vi "DAQ_DAQNodeConfigs.vi"(8 "error in":errorcluster, 10 "StreamCluster_TypeDef in":T1={"DAQ"={"ManagmentRate_Hz"=1000, "StreamRate_Hz"=10, "refDesArray"=[], "StreamRate_ms"=0, "ManagmentRate_ms"=1000}, "Modules"=[]}, 11 "DOM document in":refnum<k20>) -> (0 "error out":errorcluster={"status"=TRUE, "code"=-2633, "source"="Property Node (arg 1) in NI_XML.lvlib:Get Node Text Content.vi->CTR_ControlNodeConfigs.vi->CTR_ReadXML_Config.vi->CTRnode.vi"}, 2 "StreamCluster_TypeDef out":T1={"DAQ"={"ManagmentRate_Hz"=1000, "StreamRate_Hz"=10, "refDesArray"=[], "StreamRate_ms"=0, "ManagmentRate_ms"=1000}, "Modules"=[]}, 3 "DOM document out":refnum<k20>)   [LabVIEW 2024]
uses:
  Control/StreamCluster_TypeDef.ctl
  <vilib>/xml/Close Reference(Node).vi
  <vilib>/xml/NI_XML.lvlib
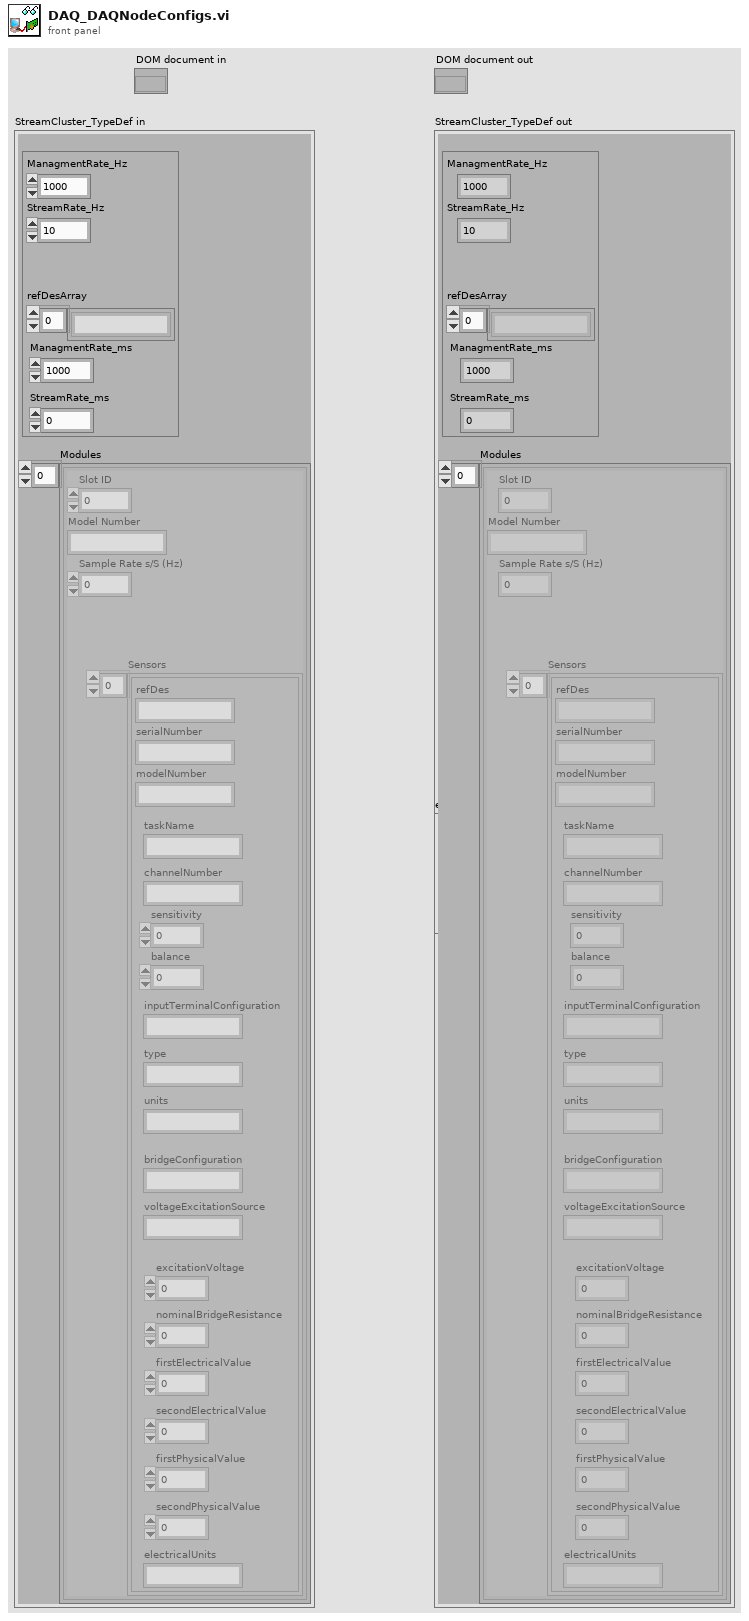
[diagram p1: front panel]
types:
  T1 = typedef "StreamCluster_TypeDef.ctl" = cluster{"DAQ":cluster{"ManagmentRate_Hz":i32, "StreamRate_Hz":i32, "refDesArray":string[], "StreamRate_ms":i32, "ManagmentRate_ms":i32}, "Modules":cluster{"Slot ID":i32, "Model Number":string, "Sample Rate s/S (Hz)":dbl, "Sensors":cluster{"refDes":string, "serialNumber":string, "modelNumber":string, "units":string, "balance":dbl, "sensitivity":dbl, "type":string, "inputTerminalConfiguration":string, "channelNumber":string, "taskName":string, "bridgeConfiguration":string, "excitationVoltage":dbl, "voltageExcitationSource":string, "nominalBridgeResistance":dbl, "firstElectricalValue":dbl, "secondElectricalValue":dbl, "firstPhysicalValue":dbl, "secondPhysicalValue":dbl, "electricalUnits":string}[]}[]}
  T2 = typedef "streamIO_states.ctl" = enum16{"Fault", "Initialize", "Stream", "Close"}
  T3 = cluster{"stream state":T2, "DAQ Node ID":i32, "Modules":cluster{"Slot ID":i32, "Model Number":string, "Sample Rate s/S (Hz)":dbl, "Sensors":cluster{"refDes":string, "serialNumber":string, "modelNumber":string, "units":string, "balance":dbl, "sensitivity":dbl, "type":string, "inputTerminalConfiguration":string, "channelNumber":string, "taskName":string, "bridgeConfiguration":string, "excitationVoltage":dbl, "voltageExcitationSource":string, "nominalBridgeResistance":dbl, "firstElectricalValue":dbl, "secondElectricalValue":dbl, "firstPhysicalValue":dbl, "secondPhysicalValue":dbl, "electricalUnits":string}[]}[], "DAQ IP Addr":string, "Restart":bool, "writer endpoint":refnum<k21>, "reader endpoint":refnum<k21>}[]
  T4 = cluster{"stream state":T2, "DAQ Node ID":i32, "Modules":cluster{"Slot ID":i32, "Model Number":string, "Sample Rate s/S (Hz)":dbl, "Sensors":cluster{"refDes":string, "serialNumber":string, "modelNumber":string, "units":string, "balance":dbl, "sensitivity":dbl, "type":string, "inputTerminalConfiguration":string, "channelNumber":string, "taskName":string, "bridgeConfiguration":string, "excitationVoltage":dbl, "voltageExcitationSource":string, "nominalBridgeResistance":dbl, "firstElectricalValue":dbl, "secondElectricalValue":dbl, "firstPhysicalValue":dbl, "secondPhysicalValue":dbl, "electricalUnits":string}[]}[], "DAQ IP Addr":string, "Restart":bool, "writer endpoint":refnum<k21>, "reader endpoint":refnum<k21>}
  T5 = cluster{"[0]":string, "[1]":string, "[2]":string, "[3]":string, "[4]":string, "[5]":string, "[6]":string, "[7]":string, "[8]":string}
  T6 = cluster{"Slot ID":i32, "Model Number":string, "Sample Rate s/S (Hz)":dbl, "Sensors":cluster{"refDes":string, "serialNumber":string, "modelNumber":string, "units":string, "balance":dbl, "sensitivity":dbl, "type":string, "inputTerminalConfiguration":string, "channelNumber":string, "taskName":string, "bridgeConfiguration":string, "excitationVoltage":dbl, "voltageExcitationSource":string, "nominalBridgeResistance":dbl, "firstElectricalValue":dbl, "secondElectricalValue":dbl, "firstPhysicalValue":dbl, "secondPhysicalValue":dbl, "electricalUnits":string}[]}[]
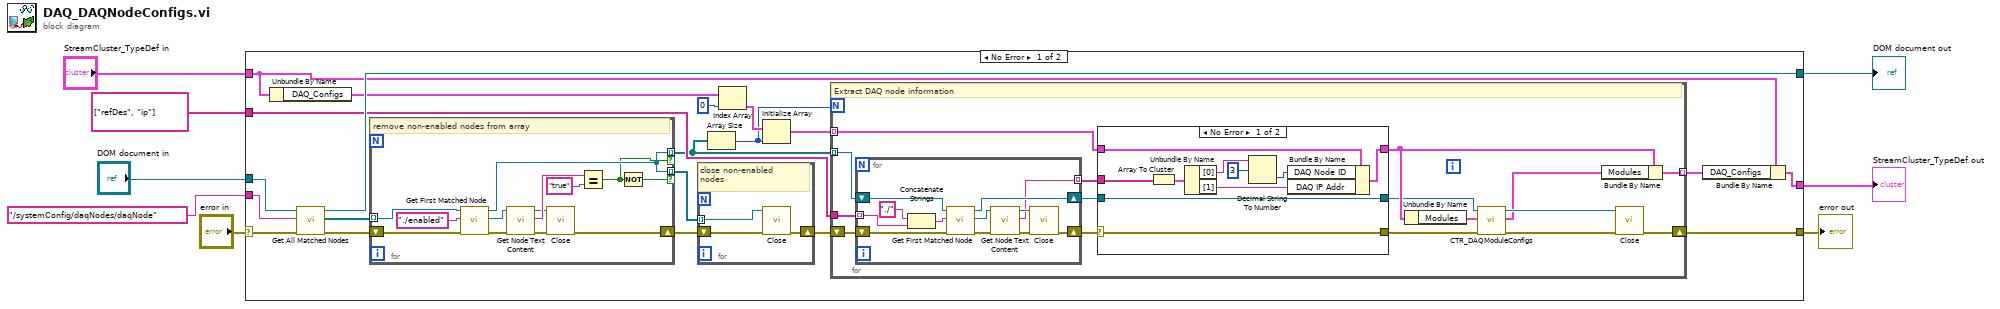
[diagram p0: block diagram]
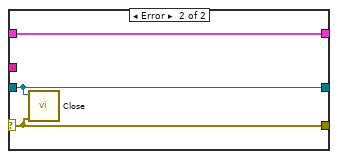
[diagram p2: hidden frame]
diagram:
  n1 = case shown="No Error" "error in" {
    selector: "error in" -> [w28 w88]
    tunnel: [w25 w88] -> w7
    tunnel: "StreamCluster_TypeDef in" -> [w24 w87]
    tunnel: [w23 w87] -> w5
    tunnel: "DOM document in" -> [w27 w86]
    tunnel: [w26 w86] -> w3
    tunnel: "/systemConfig/daqNodes/daqNode" ("XPath expression") -> [w14 _]
    tunnel: string[] ["refDes", "ip"] -> [w13 _]
    frame No Error {
      n2 = Unbundle By Name(w24) -> ("DAQ_Configs"=w22:T3)
      n3 = call <vilib>:"Get All Matched Nodes.vi"("error in (no error)"=w28, "XPath expression"=w14, "node in"=w27) -> ("error out"=w20:errorcluster, "node result array"=w19:refnum<k20>[], "node out"=w26:refnum<k20>)  [unwired: 6 in]
      n4 = for {
        shift-right: [w36] -> w16
        shift-left: w20 -> [w37]
        tunnel: w19 -> [w35] mode=indexing
        tunnel: [w34] -> w11 mode=indexing if=w32
        tunnel: [w34] -> w17 mode=indexing if=w33
        # "remove non-enabled nodes from array"
        n5 = call <vilib>:"Get First Matched Node.vi"("error in (no error)"=w37, "XPath expression"="./enabled", "node in"=w35) -> ("error out"=w40:errorcluster, "node result"=w41:refnum<k20>, "node out"=w34:refnum<k20>)  [unwired: 6 in]
        n6 = call <vilib>:"Get Node Text Content.vi"("error in (no error)"=w40, "node in"=w41) -> ("error out"=w42:errorcluster, "node text"=w44:string, "node out"=w43:refnum<k20>)  [unwired: 7 in]
        n7 = call-poly <vilib>:"Close.vi"("error in (no error)"=w42, "node"=w43) -> ("error out"=w36:errorcluster)  [unwired: 7 in]
        n8 = Equal?(x=w44, y="true" ("x")) -> (x = y?=w32:bool)
        n9 = Not(x=w32) -> (.not. x?=w33:bool)
      }
      n10 = for {
        tunnel: w17 -> [w31] mode=indexing
        shift-right: [w29] -> w15
        shift-left: w16 -> [w30]
        # "close non-enabled nodes"
        n11 = call-poly <vilib>:"Close.vi"("error in (no error)"=w30, "node"=w31) -> ("error out"=w29:errorcluster)  [unwired: 7 in]
      }
      n12 = Array Size(array=w11) -> (size(s)=w10:i32)
      n13 = Index Array(array=w22, index=0) -> (element=w12:T4)
      n14 = Initialize Array(w12, w10) -> (w18:T3)
      n15 = for {
        N: w10 -> [_]
        tunnel: w11 -> [w58] mode=indexing
        tunnel: w18 -> [w60] mode=indexing
        shift-right: [w47] -> w25
        shift-left: w15 -> [w57]
        tunnel: w13 -> [w59]
        tunnel: [w52] -> w9 mode=indexing
        # "Extract DAQ node information"
        n16 = for {
          tunnel: w59 -> [w85] mode=indexing
          shift-right: [w80] -> w53
          shift-left: w58 -> [w82]
          shift-right: [w75] -> w56
          shift-left: w57 -> [w81]
          tunnel: [w74] -> w55 mode=indexing
          n17 = Concatenate Strings("./" ("string"), w85) -> (w83:string)
          n18 = call <vilib>:"Get First Matched Node.vi"("error in (no error)"=w81, "XPath expression"=w83, "node in"=w82) -> ("error out"=w79:errorcluster, "node result"=w78:refnum<k20>, "node out"=w80:refnum<k20>)  [unwired: 6 in]
          n19 = call <vilib>:"Get Node Text Content.vi"("error in (no error)"=w79, "node in"=w78) -> ("error out"=w77:errorcluster, "node text"=w74:string, "node out"=w76:refnum<k20>)  [unwired: 7 in]
          n20 = call-poly <vilib>:"Close.vi"("error in (no error)"=w77, "node"=w76) -> ("error out"=w75:errorcluster)  [unwired: 7 out]
        }
        n21 = case shown="No Error" w56 {
          selector: w56 -> [w62 w72]
          tunnel: w53 -> [w61 w71]
          tunnel: w55 -> [w69 _]
          tunnel: w60 -> [w68 w73]
          tunnel: [w66 w73] -> w54
          tunnel: [w62 w72] -> w50
          tunnel: [w61 w71] -> w51
          frame No Error {
            n22 = Array To Cluster(array=w69) -> (cluster=w70:T5)
            n23 = Unbundle By Name(w70) -> ("[0]"=w65:string, "[1]"=w67:string)
            n24 = Decimal String To Number(string=w65, offset=u32 3 ("initial scan location")) -> (number=w63:i32)  [unwired: 1 in, 1 out]
            n25 = Bundle By Name(cluster=w68, "DAQ Node ID"=w63, "DAQ IP Addr"=w67) -> (w66:T4)
          }
          frame Error {
            n26 = call-poly <vilib>:"Close.vi"("error in (no error)"=w72, "node"=w71) -> ()  [unwired: 8 out]
          }
        }
        n27 = Unbundle By Name(w54) -> ("Modules"=w46:T6)
        n28 = call "CTR_DAQModuleConfigs.vi"("error in"=w50, "Modules in"=w46, "node in"=w51) -> ("error out"=w48:errorcluster, "Modules out"=w45:T6, "node out"=w49:refnum<k20>)  [unwired: 6 in]
        n29 = Bundle By Name(cluster=w54, "Modules"=w45) -> (w52:T4)
        n30 = call-poly <vilib>:"Close.vi"("error in (no error)"=w48, "node"=w49) -> ("error out"=w47:errorcluster)  [unwired: 7 in]
      }
      n31 = Bundle By Name(cluster=w24, "DAQ_Configs"=w9) -> (w23:T1)
    }
    frame Error {
    }
  }
  "error out" <- w7
  "DOM document out" <- w3
  "StreamCluster_TypeDef out" <- w5
